vi "GetMasterBranch.vi"(6 "error in":errorcluster, 8 "repo":string="LabVIEWforRasPi", 9 "owner":string="labviewforRaspi") -> (0 "error out":errorcluster, 4 "branch":T1)   [LabVIEW 2014, in "Raspberry Pi Compatible Compiler for LabVIEW.lvlib" / "GitHub API.lvlib"]
uses:
  GitHub API.lvlib
  TypeDefs/GitHubBranch_TD.ctl
  TypeDefs/GitHubBranchCommit_TD.ctl
  TypeDefs/GitHubCommitCommit_TD.ctl
  TypeDefs/GitHubAuthor_TD.ctl
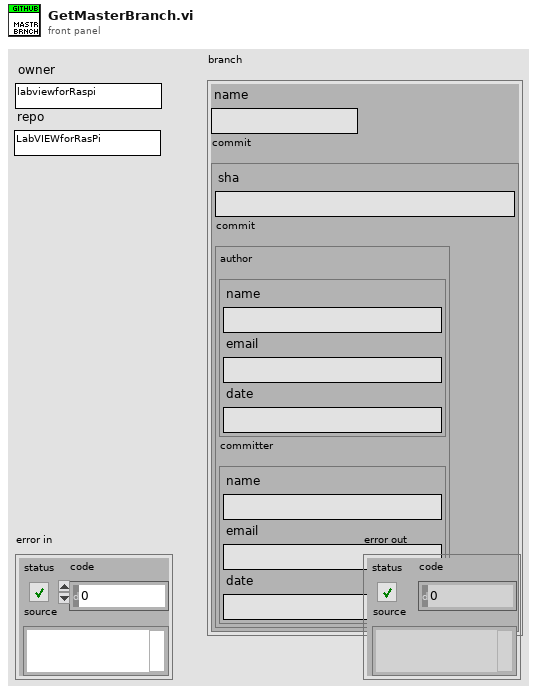
[diagram p1: front panel]
types:
  T1 = typedef "Raspberry Pi Compatible Compiler for LabVIEW.lvlib/GitHub API.lvlib/GitHubBranch_TD.ctl" = cluster{"name":string, "commit":T2}
  T2 = typedef "Raspberry Pi Compatible Compiler for LabVIEW.lvlib/GitHub API.lvlib/GitHubBranchCommit_TD.ctl" = cluster{"sha":string, "commit":T3}
  T3 = typedef "Raspberry Pi Compatible Compiler for LabVIEW.lvlib/GitHub API.lvlib/GitHubCommitCommit_TD.ctl" = cluster{"author":T4, "committer":T4}
  T4 = typedef "Raspberry Pi Compatible Compiler for LabVIEW.lvlib/GitHub API.lvlib/GitHubAuthor_TD.ctl" = cluster{"name":string, "email":string, "date":string}
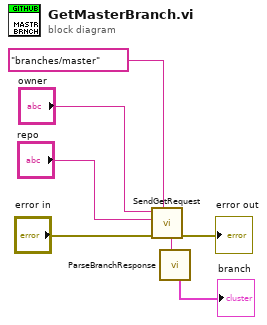
[diagram p0: block diagram]
diagram:
  n1 = call "SendGetRequest.vi"("path"="branches/master", "error in"="error in", "repo"="repo", "owner"="owner") -> ("error out"=→"error out":errorcluster, "body"=w2:string)  [unwired: 3 in, 1 out]
  n2 = call "ParseBranchResponse.vi"("body"=w2) -> ("branch"=→"branch":T1)  [unwired: 7 in, 1 out]
